vi "Connection_to_SQlite.vi"(8 "error in (no error)":errorcluster, 11 "DB_SQLite in":refnum<class "DB_SQLite.lvclass">) -> (0 "error out":errorcluster, 2 "SQlite connection":refnum<class "Connection.lvclass">, 3 "DB_SQLite out":refnum<class "DB_SQLite.lvclass">)   [LabVIEW 2015, in "DB_SQLite.lvclass"]
uses:
  DB_SQLite.lvclass
  <vilib>/drjdpowell/SQLite Library/SQL Connection/Connection.lvclass
  DB.lvclass/DB.ctl
  DB.lvclass
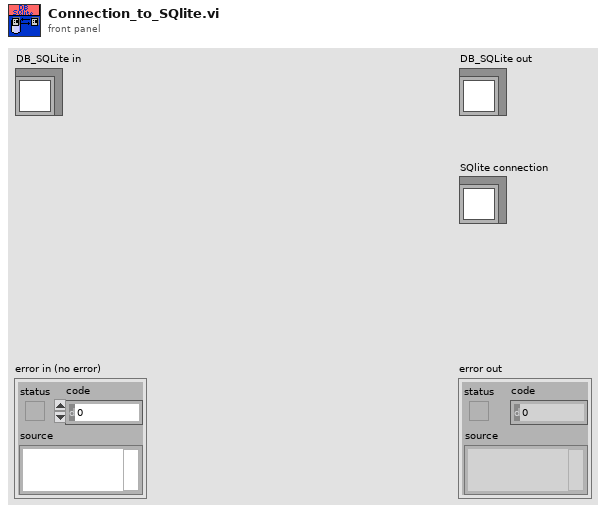
[diagram p1: front panel]
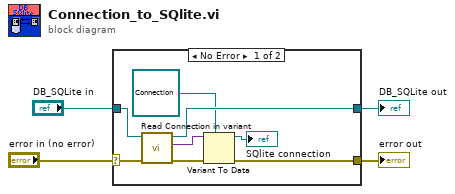
[diagram p0: block diagram]
diagram:
  n1 = case shown="No Error" "error in (no error)" {
    selector: "error in (no error)" -> [w11 w14]
    tunnel: [w8 w14] -> w3
    tunnel: [w10 w13] -> w1
    tunnel: "DB_SQLite in" -> [w12 w13]
    frame No Error {
      n2 = call "Read Connection in variant.vi"("error in (no error)"=w11, "DB in"=w12) -> ("error out"=w9:errorcluster, "Connection in variant"=w7:variant, "DB out"=w10:refnum<class "DB_SQLite.lvclass">)  [unwired: 7 in]
      n3 = Variant To Data(error in=w9, type=refnum<class "Connection.lvclass"> refnum ("SQLite Connection in"), Variant=w7) -> (data=→"SQlite connection":refnum<class "Connection.lvclass">, error out=w8:errorcluster)
    }
    frame Error {
    }
  }
  "error out" <- w3
  "DB_SQLite out" <- w1
